vi "Get BLISS_Save Server List.vi"(7 "file path (use dialog)":path, 8 "error in (no error)":errorcluster, 11 "Server Names":string[](array[string])) -> (0 "error out":errorcluster, 2 "Server Names (Dup)":string[](array[string]), 3 "File Ref Out":refnum<file>)   [LabVIEW 2020]
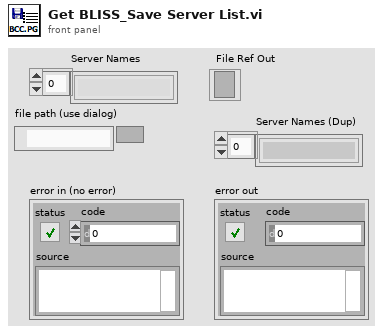
[diagram p1: front panel]
types:
  T1 = enum16{"open", "replace", "create", "open or create", "replace or create", "replace or create with confirmation"}
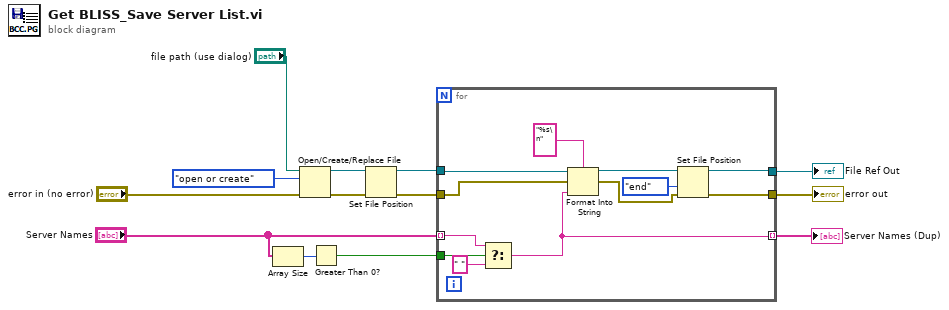
[diagram p0: block diagram]
diagram:
  n1 = Array Size(array="Server Names") -> (size(s)=w6:i32)
  n2 = Open/Create/Replace File(file path (use dialog)="file path (use dialog)", error in="error in (no error)", operation (0:open)=T1."open or create") -> (refnum out=w2:refnum<file>, error out=w4:errorcluster)  [unwired: 3 in, 1 out]
  n3 = Greater Than 0?(x=w6) -> (x > 0?=w5:bool)
  n4 = Set File Position(refnum=w2, error in=w4) -> (refnum out=w1:refnum<file>, error out=w3:errorcluster)  [unwired: 2 in]
  n5 = for {
    tunnel: [w14] -> w13 mode=indexing
    tunnel: "Server Names" -> [w16] mode=indexing
    tunnel: w1 -> [w25]
    tunnel: [w20] -> w11
    tunnel: w3 -> [w23]
    tunnel: [w18] -> w12
    tunnel: w5 -> [w17]
    n6 = Select(t=w16, s=w17, f=" ") -> (s? t:f=w14:string)
    n7 = Format Into String(format string="%s\n", initial string=w25, error in=w23, w14) -> (resulting string=w21:refnum<file>, error out=w19:errorcluster)
    n8 = Set File Position(refnum=w21, from (0:start)=enum16{"start", "end", "current"}."end", error in=w19) -> (refnum out=w20:refnum<file>, error out=w18:errorcluster)  [unwired: 1 in]
  }
  "Server Names (Dup)" <- w13
  "error out" <- w12
  "File Ref Out" <- w11
